vi "Inovance_Init_SubVI.vi"(0 "Inovance Address":T1, 11 "error in (no error)":errorcluster) -> (3 "Width":u32, 6 "Exposure":dbl, 10 "Gain":dbl, 14 "Height":u32, 15 "error out":errorcluster)   [LabVIEW 2023, in "Inovance_Camera.lvlib"]
uses:
  Inovance_Camera.lvlib
  <vilib>/userDefined/High Color/IMAQdx.ctl
  <vilib>/vision/driver/IMAQdx.llb/IMAQdx Camera Control Mode.ctl
  <vilib>/vision/driver/NI_Vision_Acquisition_Software.lvlib
  <resource>/objmgr/imaqdx.rc
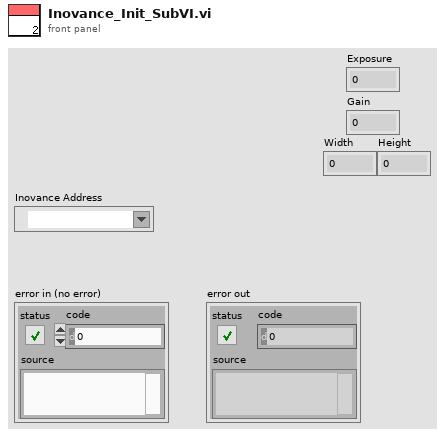
[diagram p1: front panel]
types:
  T1 = typedef "IMAQdx.ctl" = refnum<k21>
  T2 = typedef "NI_Vision_Acquisition_Software.lvlib/IMAQdx Camera Control Mode.ctl" = enum32{"Controller", "Listener"}
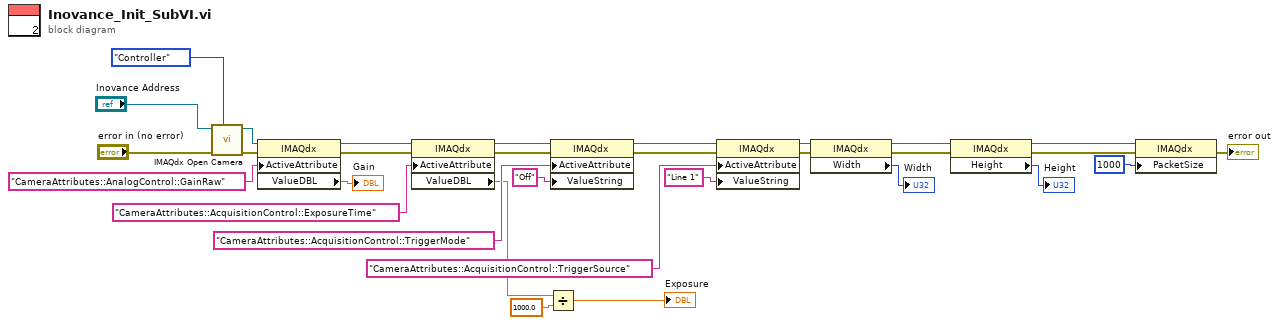
[diagram p0: block diagram]
diagram:
  n1 = call <vilib>:"IMAQdx Open Camera.vi"("Camera Control Mode"=IMAQdx_Camera_Control_Mode."Controller", "error in"="error in (no error)", "Session In"="Inovance Address") -> ("error out"=w23:errorcluster, "Session Out"=w22:T1)  [unwired: 7 in]
  n2 = property class="IMAQdx"(reference=w22, error in=w23, "ActiveAttribute"="CameraAttributes::AnalogControl::GainRaw") -> (reference out=w19:T1, error out=w20:errorcluster, "ValueDBL"=→"Gain":dbl)
  n3 = property class="IMAQdx"(reference=w19, error in=w20, "ActiveAttribute"="CameraAttributes::AcquisitionControl::ExposureTime") -> (reference out=w29:T1, error out=w31:errorcluster, "ValueDBL"=w13:dbl)
  n4 = Divide(x=w13, y=1000.0) -> (x/y=→"Exposure":dbl)
  n5 = property class="IMAQdx"(reference=w29, error in=w31, "ActiveAttribute"="CameraAttributes::AcquisitionControl::TriggerMode", "ValueString"="Off") -> (reference out=w30:T1, error out=w28:errorcluster)
  n6 = property class="IMAQdx"(reference=w30, error in=w28, "ActiveAttribute"="CameraAttributes::AcquisitionControl::TriggerSource", "ValueString"="Line 1") -> (reference out=w10:T1, error out=w1:errorcluster)
  n7 = property class="IMAQdx"(reference=w10, error in=w1) -> (reference out=w9:T1, error out=w2:errorcluster, "Width"=→"Width":u32)
  n8 = property class="IMAQdx"(reference=w9, error in=w2) -> (reference out=w5:T1, error out=w3:errorcluster, "Height"=→"Height":u32)
  n9 = property class="IMAQdx"(reference=w5, error in=w3, "PacketSize"=u32 1000) -> (error out=→"error out":errorcluster)  [unwired: 1 out]
